vi "Event-Driven State Machine - Main.vi"() -> ()   [LabVIEW 2020]
uses:
  support/State Machine Data.ctl
  support/States.ctl
  <vilib>/Utility/miscctls.llb/LVPointTypeDef.ctl
  <vilib>/DAQmx/read.llb/DAQmx Read (Analog 2D DBL NChan NSamp).vi
  <vilib>/DAQmx/write.llb/DAQmx Write (Analog DBL 1Chan 1Samp).vi
  <vilib>/DAQmx/create/channels.llb/DAQmx Create Channel (AI-Voltage-Basic).vi
  <vilib>/DAQmx/configure/timing.llb/DAQmx Timing (Sample Clock).vi
  <vilib>/DAQmx/miscellaneous.llb/DAQmx Fill In Error Info.vi
  <vilib>/Utility/file.llb/Write Delimited Spreadsheet (DBL).vi
  <vilib>/DAQmx/create/channels.llb/DAQmx Create Channel (AO-Voltage-Basic).vi
panel:
  out "RMS Results Per Channel":dbl[](array[numeric])
  out "Threshold exceeded?":bool
  in  "Acquire":bool
  in  "Samples per channel":i32=100
  in  "Sample Rate":dbl=1000.0
  in  "AI Voltage Channel":tag="PCI-6221/ai0, PCI-6221/ai2:3"
  in  "AO Voltage Channel":tag="PCI-6221/ao0"
  in  "Generate Stimulus":bool
  in  "Threshold (rms)":dbl=1.0
  in  "Clear":bool
  in  "Exit":bool
  out "Graph":dbl[][](graph)
  # "Analysis"
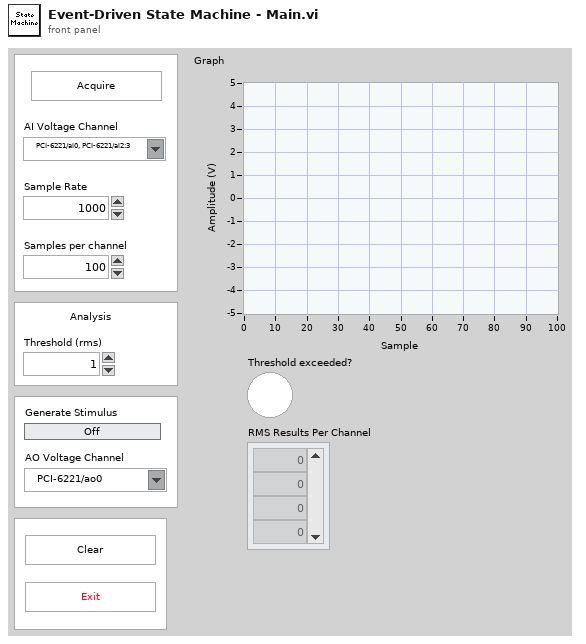
[diagram p1: front panel]
types:
  T1 = typedef "LVPointTypeDef.ctl" = cluster{"Horizontal":i16, "Vertical":i16}
  T2 = typedef "States.ctl" = enum16{"Initialize", "Wait for Event", "Acquire", "Analyze", "Log", "Clear", "Update Stimulus", "Update Graph", "Exit"}
  T3 = typedef "State Machine Data.ctl" = cluster{"Acquisition Data":dbl[][], "Stimulus Value":bool}
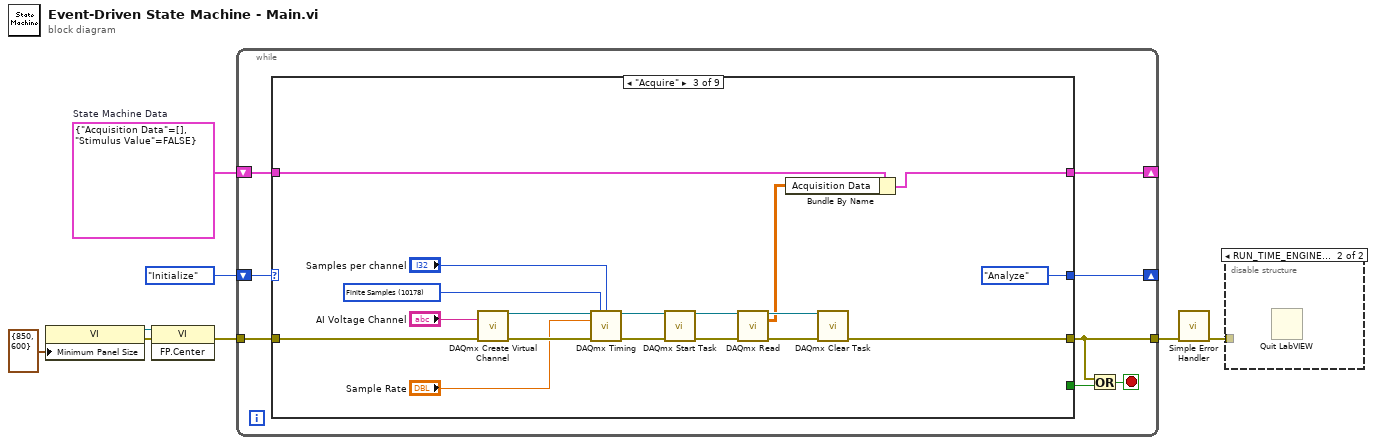
[diagram p0: block diagram]
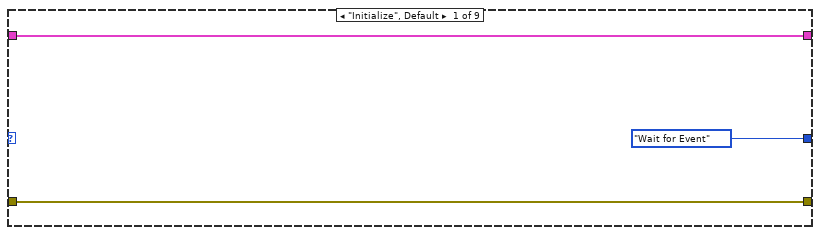
[diagram p3: hidden frame]
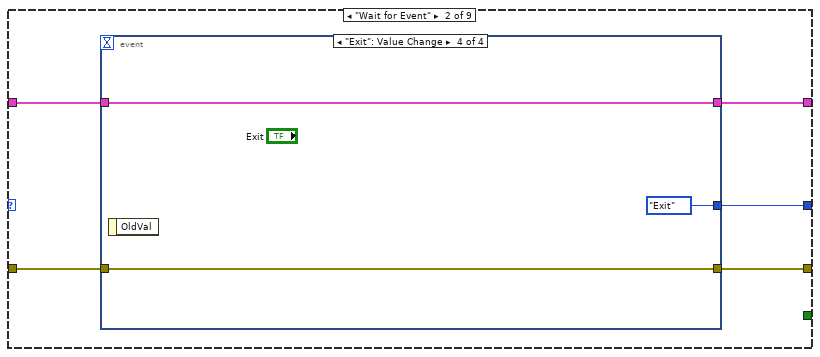
[diagram p4: hidden frame]
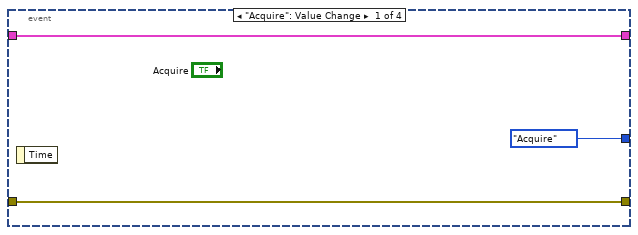
[diagram p5: hidden frame]
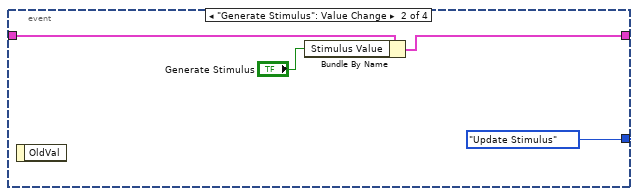
[diagram p6: hidden frame]
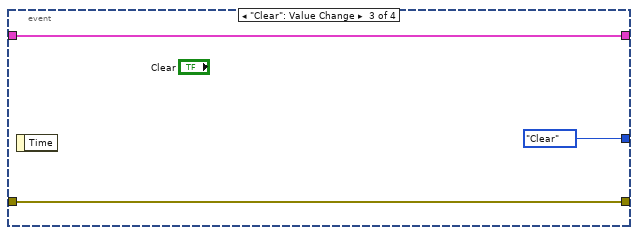
[diagram p7: hidden frame]
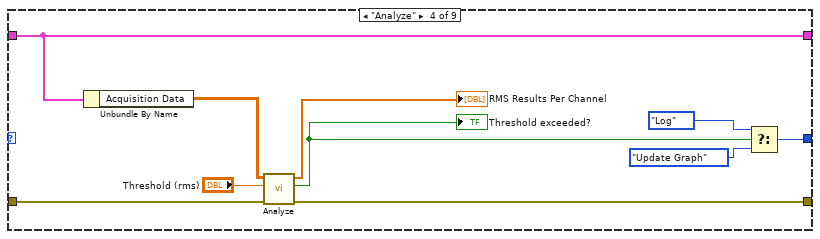
[diagram p8: hidden frame]
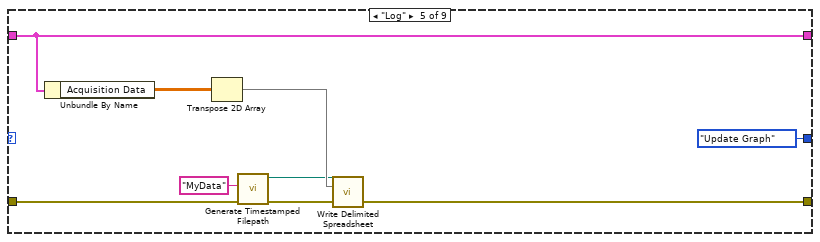
[diagram p9: hidden frame]
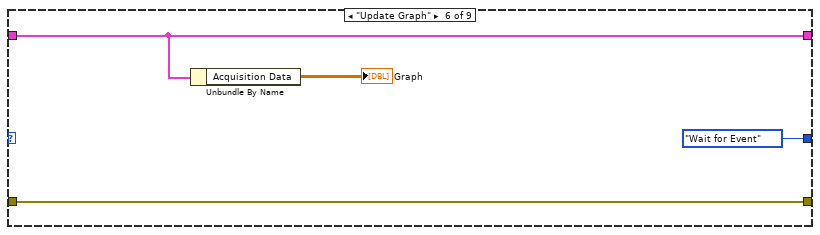
[diagram p10: hidden frame]
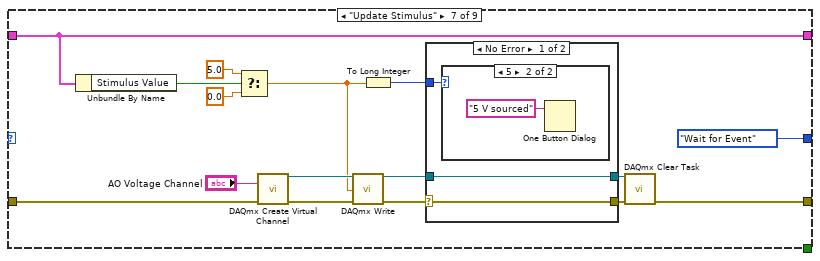
[diagram p11: hidden frame]
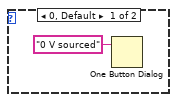
[diagram p12: hidden frame]
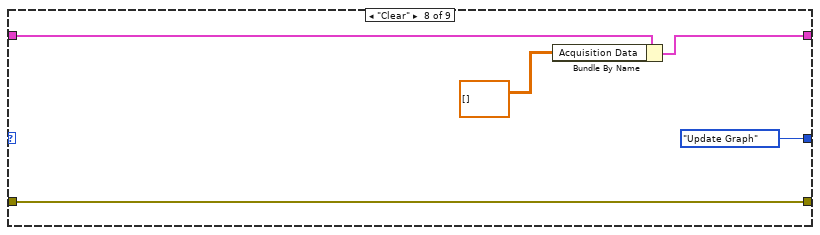
[diagram p14: hidden frame]
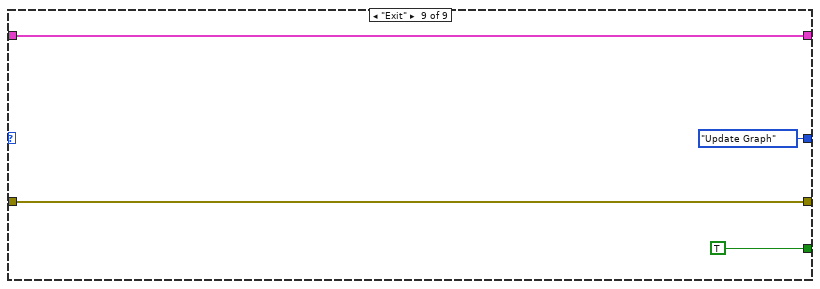
[diagram p15: hidden frame]
diagram:
  w7 = T3 {"Acquisition Data"=[], "Stimulus Value"=FALSE}  # State Machine Data
  n1 = property class="VI"("Minimum Panel Size"=T1 {"Horizontal"=850, "Vertical"=600} ("Front Panel Window:Minimum Size")) -> (reference out=w3:refnum<vi>, error out=w4:errorcluster)  [unwired: 2 in]
  n2 = invoke class="VI" method="FP.Center"(reference=w3, error in=w4) -> (error out=w5:errorcluster)  [unwired: 1 in, 2 out]
  n3 = while {
    shift-right: [w13] -> _
    shift-left: States."Initialize" ("States") -> [w16]
    shift-right: [w14] -> _
    shift-left: w7 -> [w15]
    tunnel: w5 -> [w12]
    tunnel: [w11] -> w6
    stop <- w9 stop-if-true
    n4 = case shown="\"Acquire\"" w16 {
      tunnel: w15 -> [w19 w24 w43 w65 w66 w77 w94 w105 w109]
      tunnel: [w19 w23 w39 w65 w66 w77 w94 w103 w109] -> w14
      tunnel: [States."Wait for Event" ("States") w20 States."Analyze" ("States") w57 States."Update Graph" ("States") States."Wait for Event" ("States") States."Wait for Event" ("States") States."Update Graph" ("States") States."Update Graph" ("States")] -> w13
      tunnel: w12 -> [w17 w22 w55 w62 w72 w78 w88 w106 w110]
      tunnel: [w17 w21 w41 w60 w68 w78 w89 w106 w110] -> w11
      tunnel: [_ _ _ _ _ _ _ _ TRUE] -> w10
      frame "Initialize", Default {
      }
      frame "Wait for Event" {
        n5 = event shown="[3] \"Exit\": Value Change" {
          selector: _ -> [_ _ _ _]
          dyn-events: _ -> [_ _ _ _]
          timeout: _ -> [_ _ _ _]
          tunnel: w24 -> [w26 w31 w34 w36]
          tunnel: [w26 w30 w34 w36] -> w23
          tunnel: w22 -> [w27 _ w33 w37]
          tunnel: [w27 _ w33 w37] -> w21
          tunnel: [States."Acquire" ("Enum") States."Update Stimulus" ("Enum") States."Clear" ("Enum") States."Exit" ("Enum")] -> w20
          event "Acquire": Value Change {
            n6 = event-data() -> ()  [unwired: 1 in, 1 out]
          }
          event "Generate Stimulus": Value Change {
            n7 = event-data() -> ()  [unwired: 1 in, 1 out]
            n8 = Bundle By Name(cluster=w31, "Stimulus Value"="Generate Stimulus") -> (w30:T3)
          }
          event "Clear": Value Change {
            n9 = event-data() -> ()  [unwired: 1 in, 1 out]
          }
          event "Exit": Value Change {
            n10 = event-data() -> ()  [unwired: 1 in, 1 out]
          }
        }
      }
      frame "Acquire" {
        w51 = 10178 items=["Finite Samples"=10178, "Continuous Samples"=10123, "Hardware Timed Single Point"=12522] ("sample mode")
        n11 = call-poly <vilib>:"DAQmx Create Virtual Channel.vi"("physical channels"="AI Voltage Channel", "error in"=w55) -> ("task out"=w52:refnum<k21>, "error out"=w53:errorcluster)  [unwired: 12 in]
        n12 = call-poly <vilib>:"DAQmx Timing.vi"("task/channels in"=w52, "sample mode"=w51, "samples per channel"="Samples per channel", "rate"="Sample Rate", "error in"=w53) -> ("task out"=w49:refnum<k21>, "error out"=w48:errorcluster)  [unwired: 9 in]
        n13 = call <vilib>:"DAQmx Start Task.vi"("task/channels in"=w49, "error in"=w48) -> ("task out"=w47:refnum<k21>, "error out"=w46:errorcluster)  [unwired: 12 in]
        n14 = call-poly <vilib>:"DAQmx Read.vi"("task/channels in"=w47, "error in"=w46) -> ("task out"=w45:refnum<k21>, "data"=w42:dbl[][], "error out"=w44:errorcluster)  [unwired: 11 in]
        n15 = Bundle By Name(cluster=w43, "Acquisition Data"=w42) -> (w39:T3)
        n16 = call <vilib>:"DAQmx Clear Task.vi"("task in"=w45, "error in"=w44) -> ("error out"=w41:errorcluster)  [unwired: 13 in]
      }
      frame "Analyze" {
        n17 = Unbundle By Name(w65) -> ("Acquisition Data"=w64:dbl[][])
        n18 = call "Analyze.vi"("error in (no error)"=w62, "Threshold (rms)"="Threshold (rms)", "N-Channel Data (2D DBL)"=w64) -> ("error out"=w60:errorcluster, "Threshold Exceeded?"=w56:bool, "N-Channel RMS Results"=→"RMS Results Per Channel":dbl[])  [unwired: 5 in, 1 out]
        "Threshold exceeded?" <- w56
        n19 = Select(t=States."Log" ("States"), s=w56, f=States."Update Graph" ("States")) -> (s? t:f=w57:T2)
      }
      frame "Log" {
        n20 = Unbundle By Name(w66) -> ("Acquisition Data"=w74:dbl[][])
        n21 = Transpose 2D Array(2D array=w74) -> (transposed array=w71:dbl[][])
        n22 = call "Generate Timestamped Filepath.vi"("Error In"=w72, "appended filename"="MyData") -> ("Error Out"=w69:errorcluster, "timestamped relative filepath"=w70:path)  [unwired: 8 in]
        n23 = call-poly <vilib>:"Write Delimited Spreadsheet.vi"("file path (dialog if empty)"=w70, "2D data"=w71, "error in (no error)"=w69) -> ("error out"=w68:errorcluster)  [unwired: 11 in, 1 out]
      }
      frame "Update Graph" {
        n24 = Unbundle By Name(w77) -> ("Acquisition Data"=→"Graph":dbl[][])
      }
      frame "Update Stimulus" {
        n25 = Unbundle By Name(w94) -> ("Stimulus Value"=w85:bool)
        n26 = Select(t=5.0, s=w85, f=0.0) -> (s? t:f=w84:dbl)
        n27 = call-poly <vilib>:"DAQmx Create Virtual Channel.vi"("physical channels"="AO Voltage Channel", "error in"=w88) -> ("task out"=w91:refnum<k21>, "error out"=w90:errorcluster)  [unwired: 12 in]
        n28 = call-poly <vilib>:"DAQmx Write.vi"("task/channels in"=w91, "data"=w84, "error in"=w90) -> ("task out"=w81:refnum<k21>, "error out"=w82:errorcluster)  [unwired: 10 in, 1 out]
        n29 = To Long Integer(number=w84) -> (32bit integer=w83:i32)
        n30 = case shown="No Error" w82 {
          selector: w82 -> [w95 w100]
          tunnel: w83 -> [w97 _]
          tunnel: w81 -> [w96 w101]
          tunnel: [w96 w101] -> w80
          tunnel: [w95 w100] -> w79
          frame No Error {
            n31 = case shown="5" w97 {
              frame 0, Default {
                n32 = One Button Dialog(message="0 V sourced") -> ()  [unwired: 1 in, 1 out]
              }
              frame 5 {
                n33 = One Button Dialog(message="5 V sourced") -> ()  [unwired: 1 in, 1 out]
              }
            }
          }
          frame Error {
          }
        }
        n34 = call <vilib>:"DAQmx Clear Task.vi"("task in"=w80, "error in"=w79) -> ("error out"=w89:errorcluster)  [unwired: 13 in]
      }
      frame "Clear" {
        n35 = Bundle By Name(cluster=w105, "Acquisition Data"=dbl[][] []) -> (w103:T3)
      }
      frame "Exit" {
      }
    }
    n36 = Or(x=w11, y=w10) -> (x .or. y?=w9:bool)
  }
  n37 = call <vilib>:"Simple Error Handler.vi"("error in (no error)"=w6) -> ("error out"=w1:errorcluster)  [unwired: 4 in, 4 out]
  n38 = disable-structure shown="RUN_TIME_ENGINE==True" {
    disable-tunnel: w1 -> [_ _]
    frame condition #0 (active) {
    }
    frame condition #1 {
      n39 = Quit LabVIEW() -> ()  [unwired: 1 in]
    }
  }
